vi "Zaber Home.vi"(8 "error in (no error)":errorcluster, 9 "Ir a Home":bool, 10 "Responses in":T1[](array[typedef]) {"Command" items=["Constant Speed Tracking"=8, "Echo"=55, "Error"=255, "Home"=1, "Limit Active"=9, "Manual Move Tracking"=10, "Move Absolute"=20, "Move at Constant Speed"=22, "Move Relative"=21, "Renumber"=2, "Restore Settings"=36, "Stop"=23]}, 11 "VISA Refnum in":refnum<visa-resource-name>) -> (0 "error out":errorcluster, 1 "Success?":bool, 2 "Responses out":T1[](array[typedef]) {"Command" items=["Constant Speed Tracking"=8, "Echo"=55, "Error"=255, "Home"=1, "Limit Active"=9, "Manual Move Tracking"=10, "Move Absolute"=20, "Move at Constant Speed"=22, "Move Relative"=21, "Renumber"=2, "Restore Settings"=36, "Stop"=23]}, 3 "VISA resource name out":refnum<visa-resource-name>)   [LabVIEW 2020]
doc: "Inicializa la montura Zaber, envía comando de Home y se espera hasta que llegue a home"
uses:
  <instrlib>/ZaberTSeries/ZaberTSeries.lvlib
  <instrlib>/ZaberTSeries/Public/Utility/Request.ctl
  <instrlib>/ZaberTSeries/Public/Utility/Response.ctl
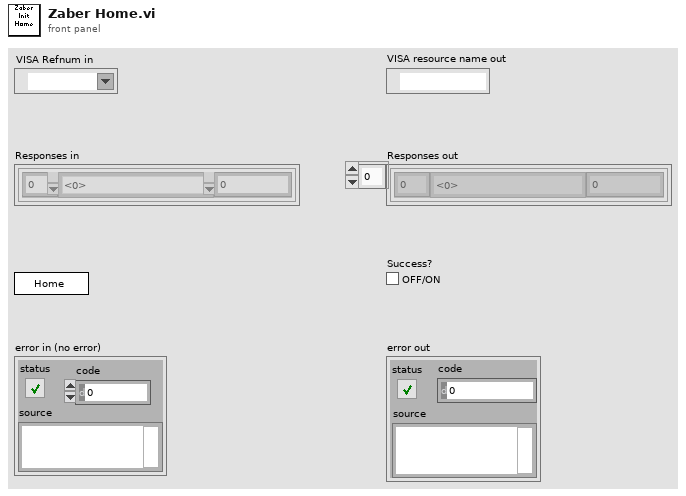
[diagram p1: front panel]
types:
  T1 = typedef "ZaberTSeries.lvlib/Response.ctl" = cluster{"Device Number":u8, "Command":u8, "Data":i32}
  T2 = typedef "ZaberTSeries.lvlib/Request.ctl" = cluster{"Device Number":u8, "Command":u8, "Data":i32, "Response Count":i32}
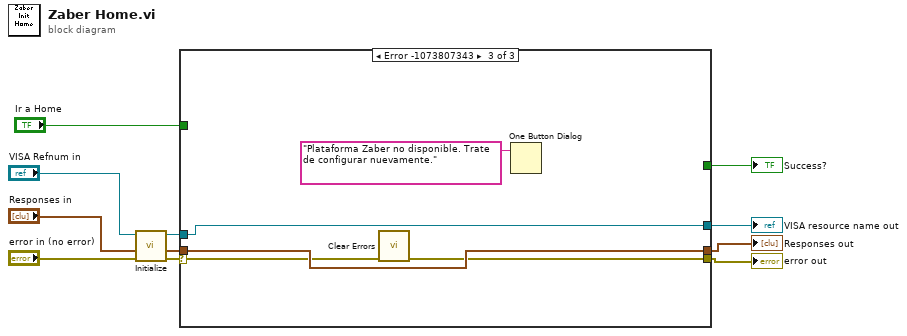
[diagram p0: block diagram]
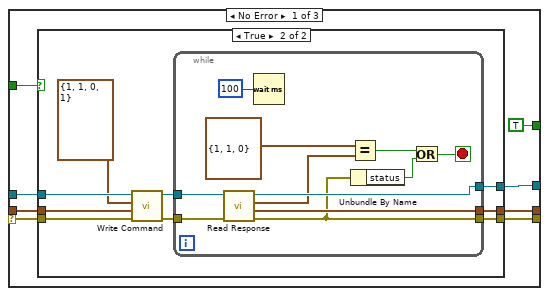
[diagram p2: hidden frame]
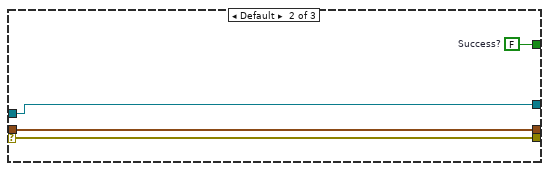
[diagram p4: hidden frame]
diagram:
  n1 = call <instrlib>:"Initialize.vi"("error in (no error)"="error in (no error)", "Responses in"="Responses in", "VISA resource name"="VISA Refnum in") -> ("error out"=w6:errorcluster, "Responses out"=w7:T1[], "VISA resource name out"=w8:refnum<visa-resource-name>)  [unwired: 6 in]
  n2 = case shown="Error -1073807343" w6 {
    selector: w6 -> [w17 w46 w49]
    tunnel: w8 -> [w19 w45 w51]
    tunnel: w7 -> [w18 w44 w50]
    tunnel: [w16 w45 w51] -> w5
    tunnel: [w15 w44 w50] -> w2
    tunnel: [w14 w46 w48] -> w4
    tunnel: "Ir a Home" -> [w13 _ _]
    tunnel: [TRUE ("Success?") w43 _] -> w1
    frame No Error {
      n3 = case shown="True" w13 {
        tunnel: w19 -> [w22 w31]
        tunnel: w18 -> [w21 w30]
        tunnel: w17 -> [w20 w27]
        tunnel: [w22 w25] -> w16
        tunnel: [w21 w24] -> w15
        tunnel: [w20 w23] -> w14
        frame False {
        }
        frame True {
          n4 = call <instrlib>:"Write Command.vi"("error in (no error)"=w27, "Responses in"=w30, "Request"=T2 {"Device Number"=1, "Command"=1, "Data"=0, "Response Count"=1}, "VISA resource name"=w31) -> ("error out"=w28:errorcluster, "VISA resource name out"=w29:refnum<visa-resource-name>)  [unwired: 5 in, 1 out]
          n5 = while {
            tunnel: w29 -> [w42]
            tunnel: w28 -> [w41]
            tunnel: [w40] -> w24
            tunnel: [w35] -> w23
            tunnel: [w38] -> w25
            stop <- w34 stop-if-true
            n6 = call <instrlib>:"Read Response.vi"("error in (no error)"=w41, "VISA resource name"=w42) -> ("error out"=w35:errorcluster, "Responses out"=w40:T1[], "Response"=w36:T1, "VISA resource name out"=w38:refnum<visa-resource-name>)  [unwired: 5 in, 1 out]
            n7 = Wait (ms)(milliseconds to wait=u32 100) -> ()  [unwired: 1 out]
            n8 = Equal?(x=T1 {"Device Number"=1, "Command"=1, "Data"=0} ("y"), y=w36) -> (x = y?=w33:bool)
            n9 = Unbundle By Name(w35) -> ("status"=w32:bool)
            n10 = Or(x=w33, y=w32) -> (x .or. y?=w34:bool)
          }
        }
      }
    }
    frame Default {
      w43 = FALSE  # Success?
    }
    frame Error {
      n11 = call <vilib>:"Clear Errors.vi"("error in (no error)"=w49) -> ("error out"=w48:errorcluster)  [unwired: 5 in, 1 out]
      n12 = One Button Dialog(message="Plataforma Zaber no disponible. Trate de configurar nuevamente.") -> ()  [unwired: 1 in, 1 out]
    }
  }
  "VISA resource name out" <- w5
  "Responses out" <- w2
  "error out" <- w4
  "Success?" <- w1
